vi "Get VI Info.vi"(1 "vi path":path=path "C:/Users/zhyang/Desktop/VIAnalyser/Rename Chassis and All Connected Modules(Template).vi") -> (0 "temporary HTML file created":path)   [LabVIEW 2016]
uses:
  <vilib>/Utility/NIReport.llb/image depth.ctl
  <vilib>/Utility/NIReport.llb/Append Report Text (str wrap).vi
  <vilib>/printing/OpenHTMLReport.llb/Open HTML Report in Browser (Refnum).vi
  <vilib>/Utility/NIReport.llb/NI_report.lvclass
  <vilib>/Utility/NIReport.llb/NI_ReportGenerationCore.lvlib
panel:
  out "error out 2":errorcluster
  out "pane view":picture
  in  "picture":picture
  out "Automatic Error Handling":bool
  out "Execution:Priority":T1(ring)
  out "Execution:Preferred Exec System":T2(ring)
  out "Execution:Inline SubVI":bool
  out "Execution:Allow Debugging":bool
  out "error out":errorcluster
  out "VI Description":string
  out "VI Name":string
  out "VI Path":path
  out "Execution:Is Reentrant":bool
  out "VI Type":T3(ring)
  out "Execution:Reentrancy Type":T4(ring)
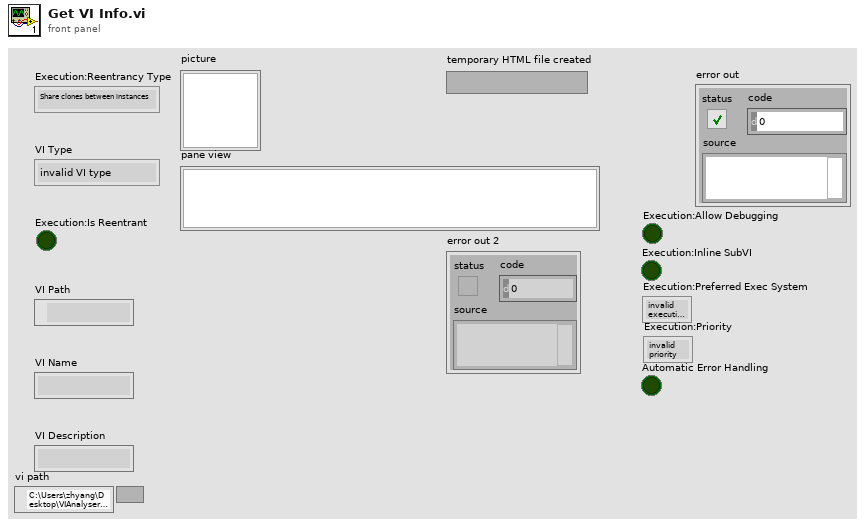
[diagram p1: front panel]
types:
  T1 = enum32{"invalid priority", "background priority", "normal priority", "above normal priority", "high priority", "time critical priority", "subroutine"}
  T2 = enum32{"invalid execution system", "user interface", "standard", "instrument i/o", "data acquisition", "other 1", "other 2", "same as caller"}
  T3 = enum32{"invalid VI type", "Standard VI", "Control VI", "Global VI", "Polymorphic VI", "Configuration VI", "SubSystem", "Facade VI", "Method VI", "Statechart Diagram VI"}
  T4 = enum16{"Share clones between instances", "Preallocate clone for each instance"}
  T5 = typedef "NI_ReportGenerationCore.lvlib/image depth.ctl" = u16
  T6 = enum16{"Standard Report", "HTML", "Word", "Excel"}
  T7 = typedef "imagedata.ctl" = cluster{"image type":i32, "image depth":i32, "image":u8[], "mask":u8[], "colors":u32[], "Rectangle":cluster{"left":i16, "top":i16, "right":i16, "bottom":i16}}
  T8 = enum16{"Invalid Wire Rule", "Required", "Recommended", "Optional", "Dynamic Dispatch"}[]
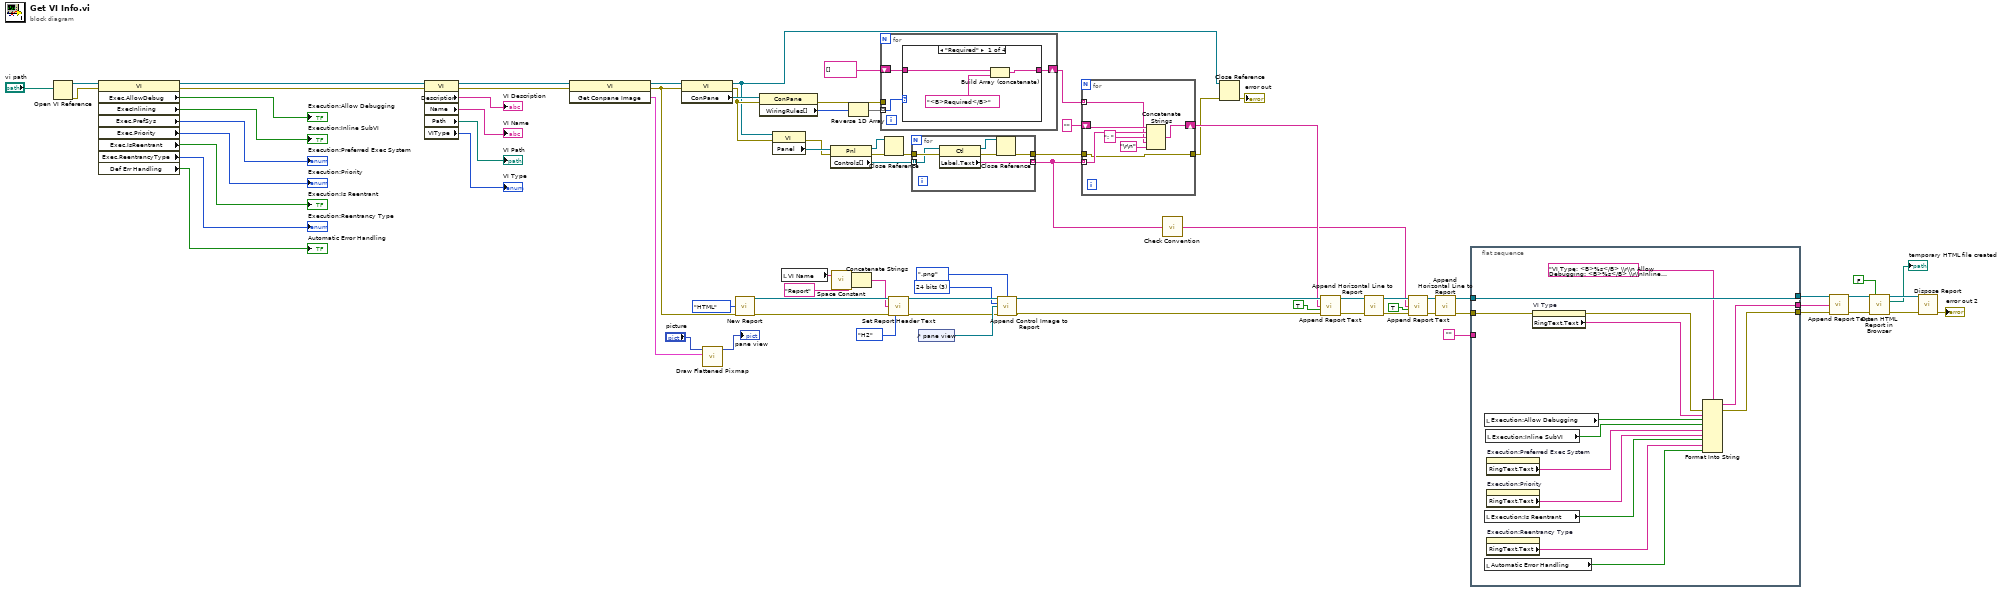
[diagram p0: block diagram]
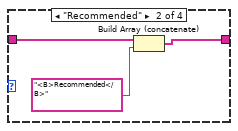
[diagram p2: hidden frame]
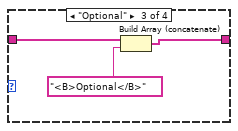
[diagram p3: hidden frame]
diagram:
  w55 = T5 3 items=["B&W", "4 bits", "8 bits", "24 bits"] ("image depth")
  n1 = Open VI Reference(vi path="vi path") -> (vi reference=w77:refnum<vi>, error out=w62:errorcluster)  [unwired: 5 in]
  n2 = property class="VI"(reference=w77, error in=w62) -> (reference out=w76:refnum<vi>, error out=w75:errorcluster, "Exec.AllowDebug"=→"Execution:Allow Debugging":bool, "ExecInlining"=→"Execution:Inline SubVI":bool, "Exec.PrefSys"=→"Execution:Preferred Exec System":T2, "Exec.Priority"=→"Execution:Priority":T1, "Exec.IsReentrant"=→"Execution:Is Reentrant":bool, "Exec.ReentrancyType"=→"Execution:Reentrancy Type":T4, "Def Err Handling"=→"Automatic Error Handling":bool)
  n3 = property class="VI"(reference=w76, error in=w75) -> (reference out=w74:refnum<vi>, error out=w73:errorcluster, "Description"=→"VI Description":string, "Name"=→"VI Name":string, "Path"=→"VI Path":path, "VIType"=→"VI Type":T3)
  n4 = invoke class="VI" method="Get Conpane Image"(reference=w74, error in=w73) -> (reference out=w44:refnum<vi>, error out=w43:errorcluster, "Get Conpane Image"=w59:T7)  [unwired: 1 in]
  n5 = property class="VI"(reference=w44, error in=w43) -> (reference out=w29:refnum<vi>, error out=w41:errorcluster, "ConPane"=w42:refnum<vi>)
  n6 = call <vilib>:"Draw Flattened Pixmap.vi"("image data"=w59, "picture"="picture") -> ("new picture"=→"pane view":picture)  [unwired: 7 in]
  n7 = call <vilib>:"New Report.vi"("report type"=T6."HTML", "error in (no error)"=w43) -> ("report out"=w53:refnum<class "NI_report.lvclass">, "error out"=w52:errorcluster)  [unwired: 12 in]
  n8 = property class="ConPane"(reference=w42, error in=w41) -> (error out=w38:errorcluster, "WiringRules[]"=w37:T8)  [unwired: 1 out]
  n9 = property class="VI"(reference=w29, error in=w41) -> (error out=w39:errorcluster, "Panel"=w40:refnum<vi>)  [unwired: 1 out]
  n10 = local read "VI Name"() -> (w7:string)
  n11 = property class="Pnl"(reference=w40, error in=w39) -> (reference out=w1:refnum<vi>, error out=w28:errorcluster, "Controls[]"=w27:refnum<vi>[])
  n12 = call <vilib>:"Space Constant.vi"() -> ("String"=w5:string)
  n13 = Reverse 1D Array(array=w37) -> (reversed array=w25:T8)
  n14 = Concatenate Strings(w7, w5, "Report" ("string")) -> (w6:string)
  n15 = for {
    tunnel: w38 -> [_]
    tunnel: w25 -> [w82] mode=indexing
    shift-right: [w80] -> w30
    shift-left: string[] [] -> [w81]
    n16 = case shown="\"Required\"" w82 {
      tunnel: w81 -> [w85 w88 w91 w92]
      tunnel: [w83 w86 w89 w92] -> w80
      frame "Required" {
        n17 = Build Array (concatenate)(w85, "<B>Required</B>") -> (w83:string[])
      }
      frame "Recommended" {
        n18 = Build Array (concatenate)(w88, "<B>Recommended</B>") -> (w86:string[])
      }
      frame "Optional" {
        n19 = Build Array (concatenate)(w91, "<B>Optional</B>") -> (w89:string[])
      }
      frame Default {
      }
    }
  }
  n20 = Close Reference(reference=w1, error in (no error)=w28) -> (error out=w2:errorcluster)
  n21 = call-dynamic "Set Report Header Text.vi"("report in"=w53, "center header text"=w6, "error in (no error)"=w52, "HTML header size"=enum16{"H1", "H2", "H3", "H4", "H5", "H6", "H7"}."H2") -> ("report out"=w56:refnum<class "NI_report.lvclass">, "error out"=w49:errorcluster)  [unwired: 10 in]
  n22 = for {
    tunnel: w2 -> [w98]
    tunnel: w27 -> [w97] mode=indexing
    tunnel: [w96] -> w24 mode=indexing
    tunnel: [w94] -> w26
    n23 = property class="Ctl"(reference=w97, error in=w98) -> (reference out=w93:refnum<vi>, error out=w95:errorcluster, "Label.Text"=w96:string)
    n24 = Close Reference(reference=w93, error in (no error)=w95) -> (error out=w94:errorcluster)
  }
  n25 = control-ref of="pane view"() -> (w50:refnum<vi>)
  n26 = call-dynamic "Append Control Image to Report.vi"("report in"=w56, "image file type (.jpg)"=enum16{".jpg", ".png"}.".png" ("image file type"), "image depth"=w55, "ctrl reference"=w50, "error in (no error)"=w49) -> ("report out"=w45:refnum<class "NI_report.lvclass">, "error out"=w18:errorcluster)  [unwired: 7 in, 2 out]
  n27 = for {
    tunnel: w24 -> [w104] mode=indexing
    tunnel: w30 -> [w102] mode=indexing
    tunnel: w26 -> [w99]
    shift-right: [w100] -> w35
    shift-left: "" -> [w105]
    tunnel: [w99] -> w32
    n28 = Concatenate Strings(w105, w104, ": " ("string"), w102, "\r\n") -> (w100:string)
  }
  n29 = call "Check Convention.vi"("terminal name array"=w24) -> ("validation result"=w21:string)
  n30 = Close Reference(reference=w29, error in (no error)=w32) -> (error out=→"error out":errorcluster)
  n31 = call-poly <vilib>:"Append Report Text.vi"("report in"=w45, "text"=w35, "append on new line? (F)"=TRUE, "error in (no error)"=w18) -> ("report out"=w47:refnum<class "NI_report.lvclass">, "error out"=w46:errorcluster)  [unwired: 8 in, 2 out]
  n32 = call-dynamic "Append Horizontal Line to Report.vi"("report in"=w47, "error in (no error)"=w46) -> ("report out"=w34:refnum<class "NI_report.lvclass">, "error out"=w22:errorcluster)  [unwired: 12 in]
  n33 = call-poly <vilib>:"Append Report Text.vi"("report in"=w34, "text"=w21, "append on new line? (F)"=TRUE, "error in (no error)"=w22) -> ("report out"=w23:refnum<class "NI_report.lvclass">, "error out"=w15:errorcluster)  [unwired: 8 in, 2 out]
  n34 = call-dynamic "Append Horizontal Line to Report.vi"("report in"=w23, "error in (no error)"=w15) -> ("report out"=w13:refnum<class "NI_report.lvclass">, "error out"=w14:errorcluster)  [unwired: 12 in]
  n35 = flat-sequence {
    tunnel: [w116] -> w17
    tunnel: [w114] -> w16
    tunnel: w14 -> [w119]
    tunnel: w13 -> [w116]
    tunnel: "" -> [_]
    tunnel: [w113] -> w10
    frame #0 {
      n36 = local read "Execution:Allow Debugging"() -> (w117:bool)
      n37 = local read "Execution:Is Reentrant"() -> (w109:bool)
      n38 = local read "Automatic Error Handling"() -> (w107:bool)
      n39 = local read "Execution:Inline SubVI"() -> (w112:bool)
      n40 = property on="Execution:Preferred Exec System" class="Enum (strict)"() -> ("RingText.Text"=w111:string)  [unwired: 2 in, 2 out]
      n41 = property on="Execution:Priority" class="Enum (strict)"() -> ("RingText.Text"=w110:string)  [unwired: 2 in, 2 out]
      n42 = property on="Execution:Reentrancy Type" class="Enum (strict)"() -> ("RingText.Text"=w108:string)  [unwired: 2 in, 2 out]
      n43 = property on="VI Type" class="Enum (strict)"(error in=w119) -> (error out=w115:errorcluster, "RingText.Text"=w118:string)  [unwired: 1 in, 1 out]
      n44 = Format Into String(format string="VI Type: <B>%s</B> \\r\\n Allow Debugging: <B>%s</B> \\r\\nInline SubVI: <B>%s</B>\\r\\n Preferred Exec System: <B>%s</B> \\r\\nPriority: <B>%s</B> \\r\\n Is Reentrant: <B>%s</B> \\r\\nReentrancy Type: <B>%s</B> \\r\\n Automatic Error Handling: <B>%s</B> \\r\\n", error in=w115, w118, w117, w112, w111, w110, w109, w108, w107) -> (resulting string=w113:string, error out=w114:errorcluster)  [unwired: 1 in]
    }
  }
  n45 = call-poly <vilib>:"Append Report Text.vi"("report in"=w17, "text"=w10) -> ("report out"=w11:refnum<class "NI_report.lvclass">)  [unwired: 10 in, 3 out]
  n46 = call-poly <vilib>:"Open HTML Report in Browser.vi"("report in"=w11, "Open in browser?"=FALSE, "error in (no error)"=w16) -> ("report out"=w33:refnum<class "NI_report.lvclass">, "temporary HTML file created"=→"temporary HTML file created":path, "error out"=w19:errorcluster)  [unwired: 10 in]
  n47 = call-dynamic "Dispose Report.vi"("report in"=w33, "error in (no error)"=w19) -> ("error out"=→"error out 2":errorcluster)  [unwired: 13 in]
